vi "Plot Position and Target in 2D.vi"(7 "bounds":T1, 9 "sub-goal":dbl[](array[numeric]), 10 "odometry data":dbl[](array[numeric]), 11 "picture in":picture) -> (3 "picture out":picture)   [LabVIEW 2011]
uses:
  <vilib>/Utility/miscctls.llb/LVBoundsTypeDef.ctl
panel:
  in  "target":cluster{"X":dbl, "Y":dbl}
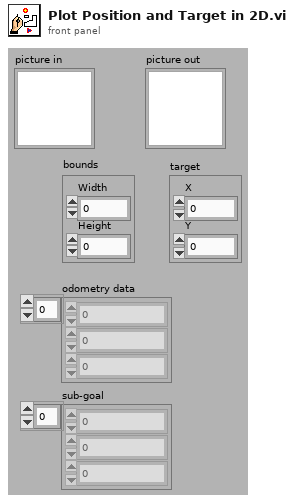
[diagram p1: front panel]
types:
  T1 = typedef "LVBoundsTypeDef.ctl" = cluster{"Width":u32, "Height":u32}
  T2 = cluster{"Width":u16, "Style":enum32{"Solid", "Dash", "Dot", "DashDot", "DashDotDot"}}
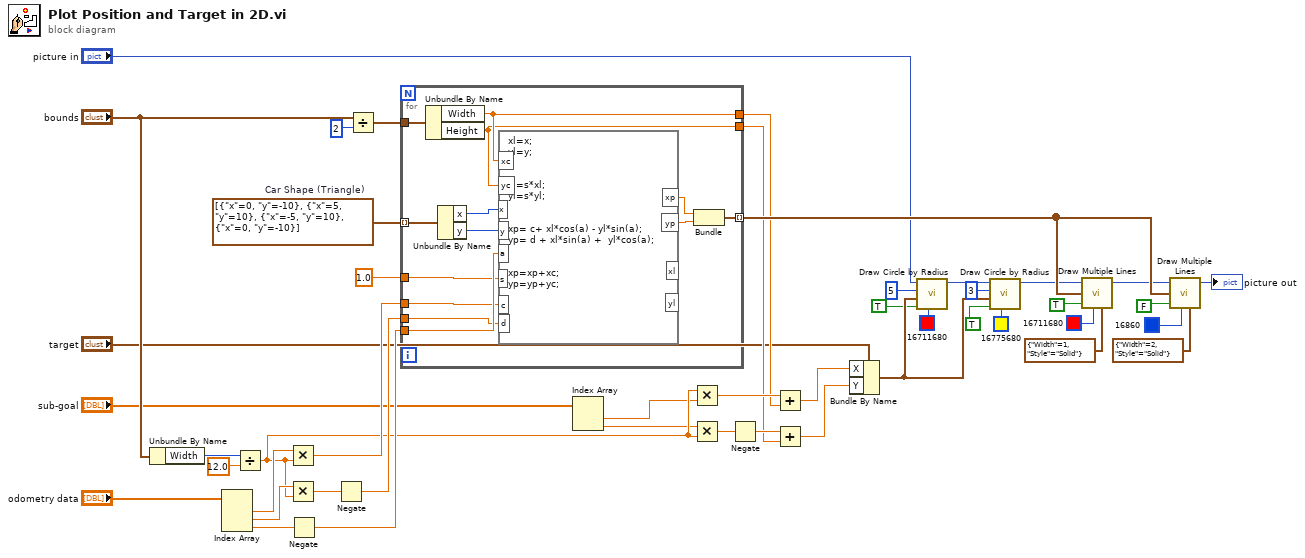
[diagram p0: block diagram]
diagram:
  w40 = cluster{"x":i16, "y":i16}[] [{"x"=0, "y"=-10}, {"x"=5, "y"=10}, {"x"=-5, "y"=10}, {"x"=0, "y"=-10}]  # Car Shape (Triangle)
  n1 = Unbundle By Name("bounds") -> ("Width"=w25:u32)
  n2 = Index Array(array="odometry data") -> (element #1=w35:dbl, element #2=w34:dbl, element #3=w33:dbl)  [unwired: 3 in]
  n3 = Divide(x=w25, y=12.0) -> (x/y=w22:dbl)
  n4 = Multiply(x=w35, y=w22) -> (x*y=w28:dbl)
  n5 = Multiply(x=w34, y=w22) -> (x*y=w29:dbl)
  n6 = Negate(x=w33) -> (-x=w30:dbl)
  n7 = Negate(x=w29) -> (-x=w24:dbl)
  n8 = Divide(x="bounds", y=2 ("x")) -> (x/y=w32:cluster{"Width":dbl, "Height":dbl})
  n9 = for {
    tunnel: w40 -> [w59] mode=indexing
    tunnel: w30 -> [w56]
    tunnel: 1.0 ("Scale") -> [w55]
    tunnel: [w54] -> w43 mode=indexing
    tunnel: w32 -> [w51]
    tunnel: w28 -> [w50]
    tunnel: w24 -> [w49]
    tunnel: [w48] -> w9
    tunnel: [w47] -> w8
    n10 = Unbundle By Name(w51) -> ("Width"=w48:dbl, "Height"=w47:dbl)
    n11 = Unbundle By Name(w59) -> ("x"=w58:i16, "y"=w57:i16)
    n12 = formula code="xl=x;\nyl=y;\n\n\nxl=s*xl;\nyl=s*yl;\n\n\nxp= c+ xl*cos(a) - yl*sin(a);\nyp= d + xl*sin(a) +  yl*cos(a);\n\n\nxp=xp+xc;\nyp=yp+yc;"("x"=w58, "y"=w57, "a"=w56, "s"=w55, "c"=w50, "d"=w49, "xc"=w48, "yc"=w47) -> ("xp"=w53:dbl, "yp"=w52:dbl)  [unwired: 2 out]
    n13 = Bundle("xp"=w53, "yp"=w52) -> (w54:cluster{"xp":dbl, "yp":dbl})  [unwired: 1 in]
  }
  n14 = Index Array(array="sub-goal") -> (element #1=w2:dbl, element #2=w1:dbl)  [unwired: 2 in]
  n15 = Multiply(x=w22, y=w2) -> (x*y=w21:dbl)
  n16 = Multiply(x=w1, y=w22) -> (x*y=w23:dbl)
  n17 = Negate(x=w23) -> (-x=w20:dbl)
  n18 = Add(x=w21, y=w9) -> (x+y=w11:dbl)
  n19 = Add(x=w20, y=w8) -> (x+y=w10:dbl)
  n20 = Bundle By Name(cluster="target", "X"=w11, "Y"=w10) -> (w19:cluster{"X":dbl, "Y":dbl})
  n21 = call <vilib>:"Draw Circle by Radius.vi"("color(black)"=u32 16711680, "fill?(F)"=TRUE, "pixel center"=w19, "radius"=i16 5, "picture"="picture in") -> ("new picture"=w18:picture)  [unwired: 6 in]
  n22 = call <vilib>:"Draw Circle by Radius.vi"("color(black)"=u32 16775680, "fill?(F)"=TRUE, "pixel center"=w19, "radius"=i16 3, "picture"=w18) -> ("new picture"=w6:picture)  [unwired: 6 in]
  n23 = call <vilib>:"Draw Multiple Lines.vi"("picture"=w6, "line endpoints"=w43, "fill?(F)"=TRUE, "color(black)"=u32 16711680, "pen"=T2 {"Width"=1, "Style"=enum."Solid"}) -> ("new picture"=w42:picture)  [unwired: 4 in]
  n24 = call <vilib>:"Draw Multiple Lines.vi"("picture"=w42, "line endpoints"=w43, "fill?(F)"=FALSE, "color(black)"=u32 16860, "pen"=T2 {"Width"=2, "Style"=enum."Solid"}) -> ("new picture"=→"picture out":picture)  [unwired: 4 in]
